vi "Clear stop flag.vi"(8 "error in (no error)":errorcluster, 11 "Motor in":refnum<class "Motor.lvclass">) -> (0 "error out":errorcluster, 3 "Motor out":refnum<class "Motor.lvclass">)   [LabVIEW 2018, in "Motor.lvclass"]
uses:
  Motor.lvclass
  Motor.lvclass/Motor.ctl
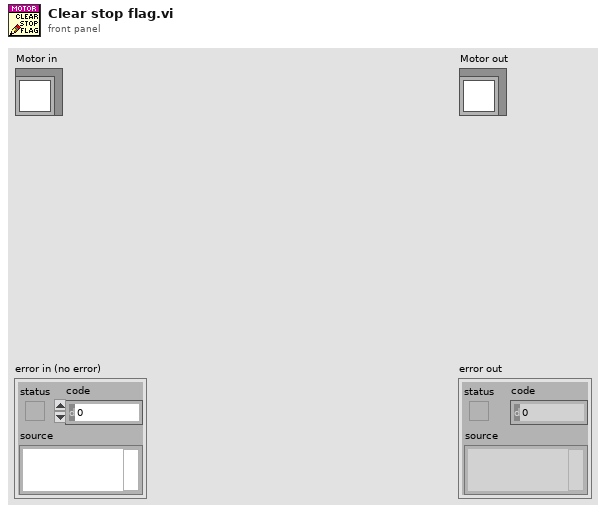
[diagram p1: front panel]
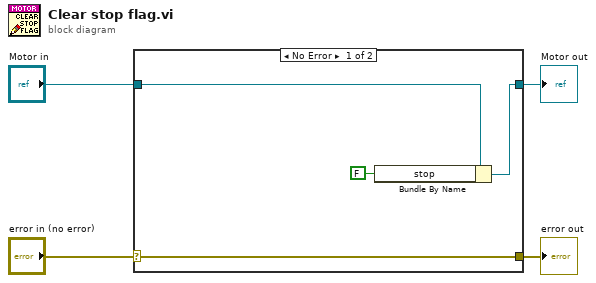
[diagram p0: block diagram]
diagram:
  n1 = case shown="No Error" "error in (no error)" {
    selector: "error in (no error)" -> [w8 w9]
    tunnel: [w8 w9] -> w3
    tunnel: [w6 w10] -> w1
    tunnel: "Motor in" -> [w7 w10]
    frame No Error {
      n2 = Bundle By Name(cluster=w7, "stop"=FALSE ("command in.stop")) -> (w6:refnum<class "Motor.lvclass">)
    }
    frame Error {
    }
  }
  "error out" <- w3
  "Motor out" <- w1
